vi "Stop.vi"(8 "error in (no error)":errorcluster, 11 "Multimeter in":refnum<class "Multimeter.lvclass">) -> (0 "error out":errorcluster, 3 "Multimeter out":refnum<class "Multimeter.lvclass">)   [LabVIEW 2015, in "Multimeter.lvclass"]
uses:
  Multimeter.lvclass
  Device.lvclass
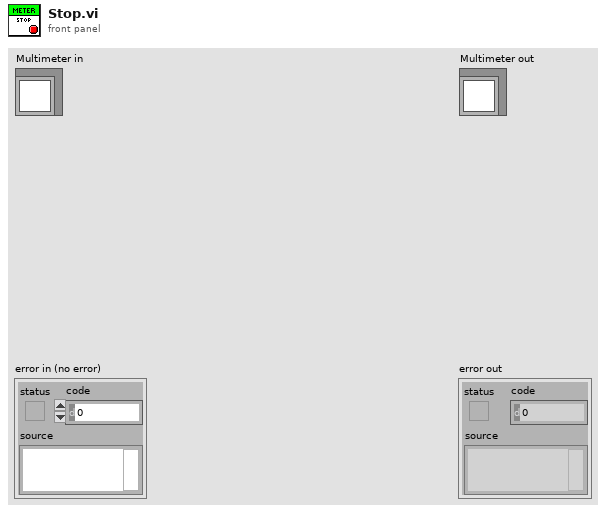
[diagram p1: front panel]
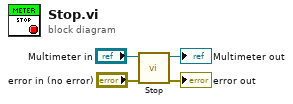
[diagram p0: block diagram]
diagram:
  n1 = call-parent "Stop.vi"("error in (no error)"="error in (no error)", "Device in"="Multimeter in") -> ("error out"=→"error out":errorcluster, "Device out"=→"Multimeter out":refnum<class "Multimeter.lvclass">)  [unwired: 8 in]
